vi "edit io channel.vi"(6 "user event":T2, 7 "Properties:instance identifier":string, 8 "error in":errorcluster, 9 "line":T1, 10 "engine configuration in":refnum<class "engine configuration.lvclass">, 11 "tag bus configurable plugin module configuration in":refnum<class "tag bus configurable plugin module configuration.lvclass">) -> (0 "error out":errorcluster, 2 "engine configuration":refnum<class "engine configuration.lvclass">, 3 "tag bus configurable plugin module configuration out":refnum<class "tag bus configurable plugin module configuration.lvclass">)   [LabVIEW 2013, in "tag bus configurable plugin editor node.lvclass"]
uses:
  tag bus configurable plugin editor node.lvclass
  <vilib>/CEF_TreeControl/Node/UserEventRef.ctl
  <vilib>/CEF_TreeControl/Controls/EventCluster.ctl
  <vilib>/NI/Module Execution Interface/Engine Configuration/engine configuration.lvclass
  module/configuration/tag bus configurable plugin module configuration.lvclass
  table line.ctl
  <vilib>/NI/Tag Bus Module Framework/channel/TBM channel.lvclass
  <vilib>/NI/Tag Bus/tag/tag descriptor.lvclass/tag descriptor.ctl
  <vilib>/CEF_TreeControl/NISE_CEF_TreeControl.lvlib
  <vilib>/NI/Tag Bus/tag/tag descriptor.lvclass
  <vilib>/CEF_TreeControl/Node/NISE_CEF_Node.lvclass
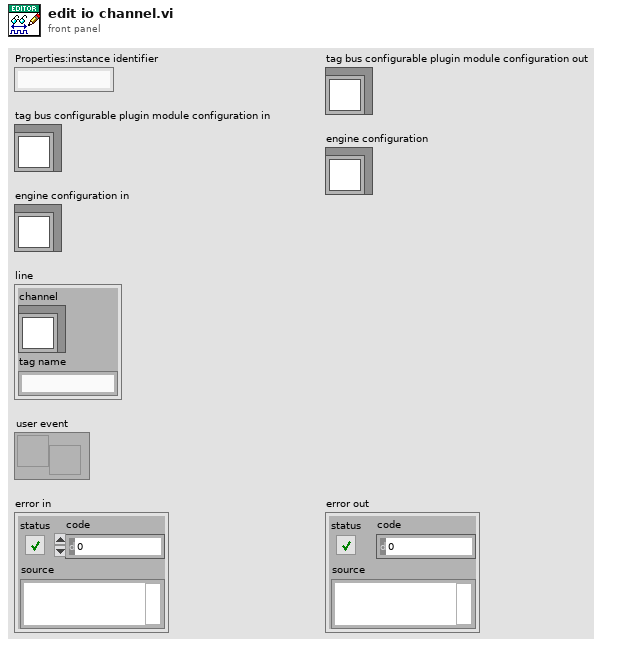
[diagram p1: front panel]
types:
  T1 = typedef "tag bus configurable plugin editor node.lvclass/table line.ctl" = cluster{"channel":refnum<class "TBM channel.lvclass">, "tag name":string}
  T2 = typedef "NISE_CEF_Node.lvclass/UserEventRef.ctl" = refnum<user-event>
  T3 = typedef "NISE_CEF_TreeControl.lvlib/EventCluster.ctl" = cluster{"command":string, "data":string}
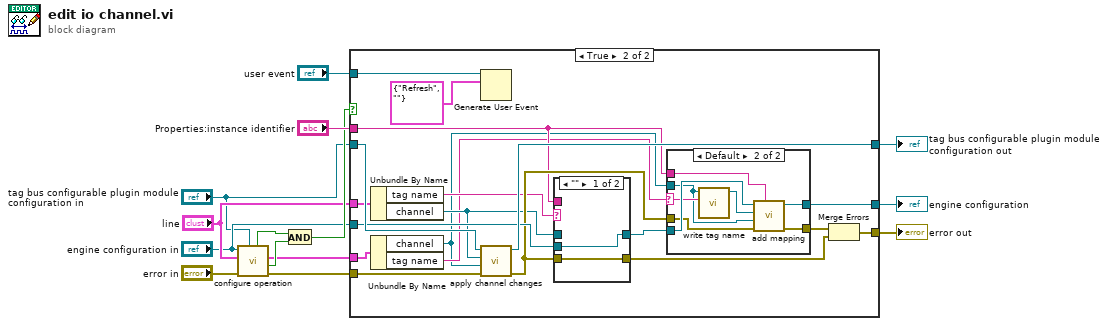
[diagram p0: block diagram]
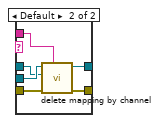
[diagram p4: hidden frame]
diagram:
  n1 = call "configure operation.vi"("tag bus configurable plugin module configuration"="tag bus configurable plugin module configuration in", "error in"="error in", "line item in"="line", "engine configuration"="engine configuration in") -> ("error out"=w5:errorcluster, "success"=w9:bool, "line item out"=w6:T1, "changed"=w8:bool)  [unwired: 4 in]
  n2 = And(x=w8, y=w9) -> (x .and. y?=w10:bool)
  n3 = case shown="True" w10 {
    tunnel: [w16 w24] -> w3
    tunnel: [w17 w27] -> w12
    tunnel: "engine configuration in" -> [w17 w29]
    tunnel: w5 -> [w16 w33]
    tunnel: w6 -> [_ w35]
    tunnel: "line" -> [_ w34]
    tunnel: "tag bus configurable plugin module configuration in" -> [w15 w36]
    tunnel: [w15 w30] -> w11
    tunnel: "Properties:instance identifier" -> [_ w20]
    tunnel: "user event" -> [_ w31]
    frame False {
    }
    frame True {
      n4 = Unbundle By Name(w34) -> ("tag name"=w22:string, "channel"=w21:refnum<class "TBM channel.lvclass">)
      n5 = Unbundle By Name(w35) -> ("channel"=w18:refnum<class "TBM channel.lvclass">, "tag name"=w19:string)
      n6 = Generate User Event(user event=w31, event data cluster=T3 {"command"="Refresh", "data"=""} ("event data")) -> ()  [unwired: 2 in, 2 out]
      n7 = call "apply channel changes.vi"("error in"=w33, "new channel"=w18, "old channel"=w21, "tag bus configurable plugin module configuration in"=w36) -> ("error out"=w23:errorcluster, "tag bus configurable plugin module configuration out"=w30:refnum<class "tag bus configurable plugin module configuration.lvclass">)  [unwired: 6 in]
      n8 = case shown="\"\"" w22 {
        tunnel: w20 -> [_ w54]
        tunnel: w29 -> [w48 w53]
        tunnel: [w48 w52] -> w28
        tunnel: [w47 w51] -> w26
        tunnel: w23 -> [w47 w50]
        tunnel: w21 -> [_ w49]
        frame "" {
        }
        frame Default {
          n9 = call <vilib>:"delete mapping by channel.vi"("owner ID"=w54, "error in"=w50, "channel"=w49, "engine configuration in"=w53) -> ("error out"=w51:errorcluster, "engine configuration out"=w52:refnum<class "engine configuration.lvclass">)  [unwired: 6 in]
        }
      }
      n10 = case shown="Default" w19 {
        selector: w19 -> [_ w40]
        tunnel: w28 -> [w38 w46]
        tunnel: [w38 w45] -> w27
        tunnel: [w37 w44] -> w25
        tunnel: w23 -> [w37 w43]
        tunnel: w20 -> [_ w42]
        tunnel: w18 -> [_ w39]
        frame "" {
        }
        frame Default {
          n11 = call <vilib>:"write tag name.vi"("name"=w40, "system tag in"=w39) -> ("system tag out"=w41:refnum<class "TBM channel.lvclass">)  [unwired: 8 in, 1 out]
          n12 = call <vilib>:"add mapping.vi"("owner ID"=w42, "error in"=w43, "channel"=w39, "tag descriptor"=w41, "engine configuration"=w46) -> ("error out"=w44:errorcluster, "engine configuration out"=w45:refnum<class "engine configuration.lvclass">)  [unwired: 5 in]
        }
      }
      n13 = Merge Errors(w25, w26) -> (w24:errorcluster)
    }
  }
  "engine configuration" <- w12
  "tag bus configurable plugin module configuration out" <- w11
  "error out" <- w3
